vi "Read_PHD_FromSIS_2020-11-06.vi"(7 "file path (dialog if empty)":path) -> (0 "PHDHist":T2(graph), 1 "Average SIS from Filtered Data":cluster{dbl[], dbl[]}(graph), 3 "Mean_mVns":dbl, 4 "Median_mVns":dbl, 5 "PHDValues":dbl[](array[numeric]), 6 "SIS Data":T1)   [LabVIEW 2018]
uses:
  <vilib>/Analysis/NI_AALPro.lvlib
  <vilib>/Analysis/NI_AALBase.lvlib
panel:
  out "FWHM":dbl
  out "Max":dbl
  out "PulseHeightRes":dbl
  out "lowercase file extension":string
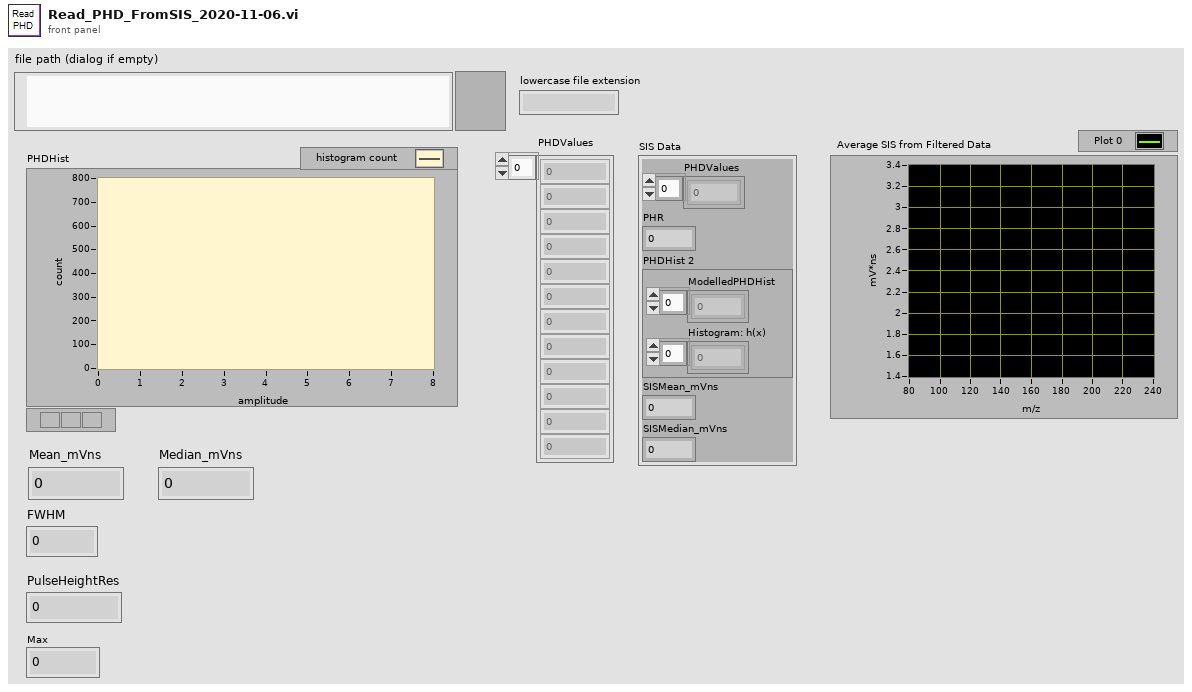
[diagram p1: front panel]
types:
  T1 = cluster{"PHDValues":dbl[], "PHR":dbl, "PHDHist 2":cluster{"ModelledPHDHist":dbl[], "Histogram: h(x)":i32[]}, "SISMean_mVns":dbl, "SISMedian_mVns":dbl}
  T2 = cluster{"X Values":dbl[], "Histogram: h(x)":i32[]}
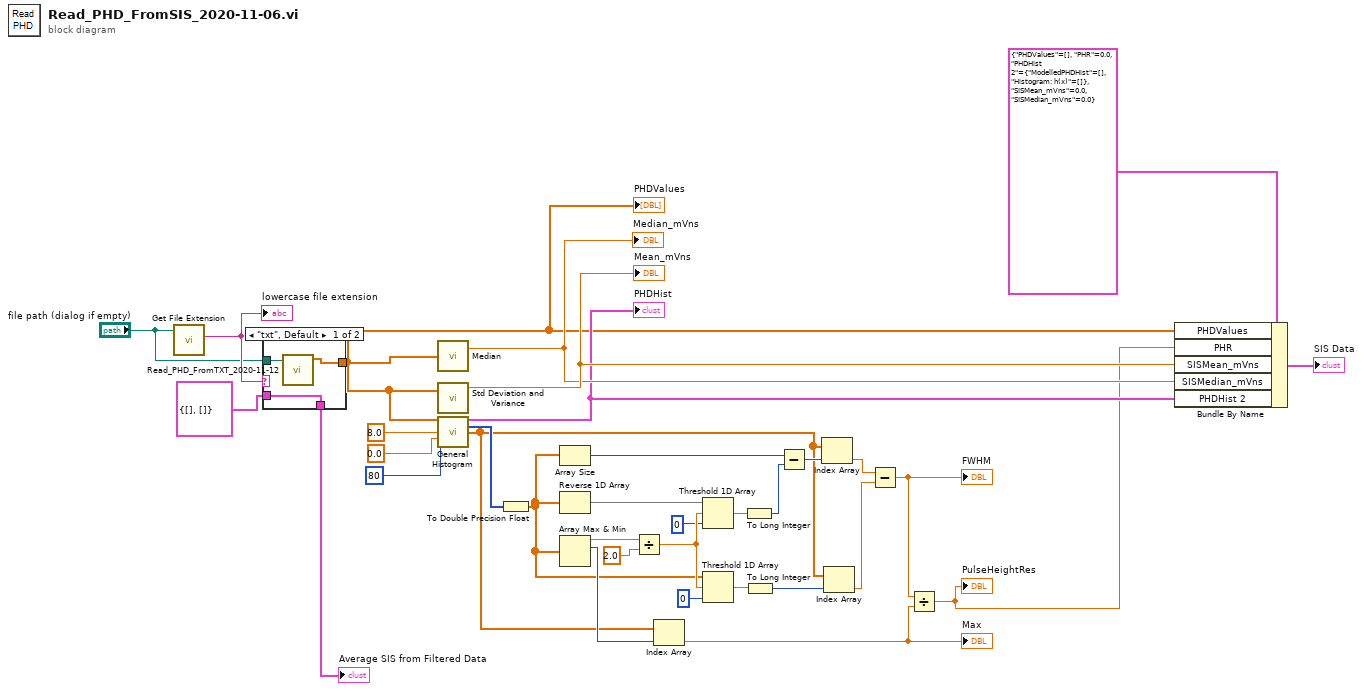
[diagram p0: block diagram]
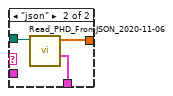
[diagram p2: hidden frame]
diagram:
  n1 = call <vilib>:"Get File Extension.vi"("file"="file path (dialog if empty)") -> ("lowercase file extension"=w25:string)  [unwired: 6 in, 4 out]
  "lowercase file extension" <- w25
  n2 = case shown="\"txt\", Default" w25 {
    tunnel: "file path (dialog if empty)" -> [w37 w40]
    tunnel: [w36 w39] -> w23
    tunnel: [w35 w38] -> w1
    tunnel: cluster{dbl[], dbl[]} {[], []} ("Average SIS from Filtered Data") -> [w35 _]
    frame "txt", Default {
      n3 = call "Read_PHD_FromTXT_2020-11-12.vi"("file path (dialog if empty)"=w37) -> ("PHDValues"=w36:dbl[])  [unwired: 10 in]
    }
    frame "json" {
      n4 = call "Read_PHD_FromJSON_2020-11-06.vi"("file (use dialog)"=w40) -> ("Average SIS from Filtered Data"=w38:cluster{dbl[], dbl[]}, "Filtered SIS Hist in mV-ns"=w39:dbl[])  [unwired: 9 in]
    }
  }
  "PHDValues" <- w23
  "Average SIS from Filtered Data" <- w1
  n5 = call <vilib>:"Median.vi"("X"=w23) -> ("median"=w31:dbl)  [unwired: 1 out]
  "Median_mVns" <- w31
  n6 = call <vilib>:"Std Deviation and Variance.vi"("X"=w23) -> ("mean"=w32:dbl)  [unwired: 1 in, 2 out]
  "Mean_mVns" <- w32
  n7 = call <vilib>:"General Histogram.vi"("X"=w23, "max"=8.0, "min"=0.0, "# bins"=80) -> ("Histogram Graph"=w30:T2, "Histogram"=w34:i32[], "Axis"=w4:dbl[])  [unwired: 7 in, 2 out]
  "PHDHist" <- w30
  n8 = To Double Precision Float(number=w34) -> (double precision float=w5:dbl[])
  n9 = Array Size(array=w5) -> (size(s)=w11:i32)
  n10 = Reverse 1D Array(array=w5) -> (reversed array=w14:dbl[])
  n11 = Array Max & Min(array=w5) -> (max value=w8:dbl, max index (indices)=w10:i32)  [unwired: 2 out]
  n12 = Divide(x=w8, y=2.0) -> (x/y=w15:dbl)
  n13 = Index Array(array=w4, index=w10) -> (element=w6:dbl)
  "Max" <- w6
  n14 = Threshold 1D Array(1:0 ("start index (0)"), 2:w15, 3:w14) -> (0:w18:dbl)
  n15 = Threshold 1D Array(1:0 ("start index (0)"), 2:w15, 3:w5) -> (0:w20:dbl)
  n16 = To Long Integer(number=w18) -> (32bit integer=w12:i32)
  n17 = To Long Integer(number=w20) -> (32bit integer=w19:i32)
  n18 = Subtract(x=w11, y=w12) -> (x-y=w7:i32)
  n19 = Index Array(array=w4, index=w7) -> (element=w17:dbl)
  n20 = Index Array(array=w4, index=w19) -> (element=w16:dbl)
  n21 = Subtract(x=w17, y=w16) -> (x-y=w9:dbl)
  "FWHM" <- w9
  n22 = Divide(x=w9, y=w6) -> (x/y=w3:dbl)
  "PulseHeightRes" <- w3
  n23 = Bundle By Name(cluster=T1 {"PHDValues"=[], "PHR"=0.0, "PHDHist 2"={"ModelledPHDHist"=[], "Histogram: h(x)"=[]}, "SISMean_mVns"=0.0, "SISMedian_mVns"=0.0} ("input cluster"), "PHDValues"=w23, "PHR"=w3, "SISMean_mVns"=w32, "SISMedian_mVns"=w31, "PHDHist 2"=w30) -> (→"SIS Data":T1)
